vi "dfd_QMF Lattice Synthesis Bank with State (Array).vi"(6 "state in":cluster{"state":dbl[]}[](array[cluster]), 8 "error in (no error)":errorcluster, 9 "filter bank":T1 {"mBank_Type" items=["Uniform", "Non-Uniform"]; "mBank_Filters"."mMRate_SumWl" min=1 max=32 step=1; "mBank_Filters"."mMRate_InputIwl" min=1 max=32 step=1; "mBank_Filters"."mMRate_GainWl" min=1 max=32 step=1; "mBank_Filters"."mMRate_OutputWl" min=1 max=32 step=1; "mBank_Filters"."mMRate_InputWl" min=1 max=32 step=1; "mBank_Filters"."mMRate_CoefWl" min=1 max=32 step=1; "mBank_Filters"."mMRate_Mode" items=["Default"=-1, "No Rate Change"=0, "Interpolation"=1, "Decimation"=2, "Interpolated"=3, "Rational"=4]}, 10 "x 2":dbl[](array[numeric]) format="%.2f", 11 "x1":dbl[](array[numeric]) format="%.2f") -> (0 "error out":errorcluster, 3 "y1":dbl[](array[numeric]) format="%.2f", 4 "state out":cluster{dbl[]}[](array[cluster]))   [LabVIEW 2017, in "NI_DigFilter_FilterBank.lvlib"]
uses:
  <vilib>/addons/Digital Filter Design/NI_DigFilter_FilterBank.lvlib
  <vilib>/addons/Digital Filter Design/FilterBank.llb/Object/DFD Bank Obj.ctl
  <vilib>/addons/Digital Filter Design/_Objects.llb/DFD Multirate Filter Obj.ctl
  <vilib>/addons/Digital Filter Design/_Objects.llb/DFD Multirate Mode.ctl
  <vilib>/addons/Digital Filter Design/_Objects.llb/DFD Coef Norm Type.ctl
  <vilib>/addons/Digital Filter Design/_Objects.llb/DFD Round-off Mode.ctl
  <vilib>/addons/Digital Filter Design/_Objects.llb/DFD FXP MRate Multiply Mode.ctl
  <vilib>/addons/Digital Filter Design/FilterBank.llb/Object/DFD Filter Bank Processing Method.ctl
  <vilib>/addons/Digital Filter Design/FilterBank.llb/Object/DFD Filter Bank Type.ctl
  <vilib>/addons/Digital Filter Design/_Misc.llb/dfd_Error Cluster From Error Code (Scalar).vi
  <vilib>/addons/Digital Filter Design/NI_DigFilterLicensed.lvlib
  <resource>/LVDFD.dll
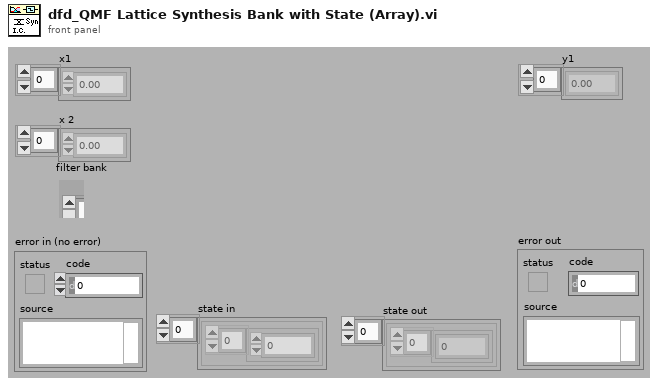
[diagram p1: front panel]
types:
  T1 = typedef "NI_DigFilter_FilterBank.lvlib/DFD Bank Obj.ctl" = cluster{"mBank_Filters":T2[], " mBank_#Bands":i32, "mBank_ProcMethod":T7, "mBank_Coeffs":dbl[], "mBank_Gain":dbl, "mBank_Type":T8}
  T2 = typedef "NI_DigFilterLicensed.lvlib/DFD Multirate Filter Obj.ctl" = cluster{"mMRate_Structure":enum16{"CIC", "FIR", "IIR", "Lattice"}, "mMRate_Mode":T3, "mMRate_Factor":i32, "mMRate_FIRParams":cluster{"mMRate_FIR_H":dbl[], "mMRate_FIR_IsNyquist?":bool, "mMRate_FIR_IsSymmetric?":bool}, "mMRate_CICParams":cluster{"mMRate_CIC_#Stage":i32, "mMRate_CIC_Lag":i32, "mMRate_CIC_Type":enum16{"Lowpass", "Highpass"}}, "mMRate_Order":i32, "mMRate_Version":string, "mMRate_Comments":string, "mMRate_RationalFactor":cluster{"mMRate_L":i32, "mMRate_M":i32}, "mMRate_Fs":dbl, "mMRate_Quantized?":bool, "mMRate_QFilterGain":dbl, "mMRate_CoefWl":i16, "mMRate_Scaling":cluster{"mMRate_ScaleByPowerOf2?":bool, "mMRate_ScaleType":T4}, "mMRate_InputWl":i16, "mMRate_OutputWl":i16, "mMRate_OutputMode":T5, "mMRate_MultMode":T6, "mMRate_BitPruning":bool, "mMRate_GainWl":i16, "mMRate_OutputFwl":i16, "mMRate_SumIwl":i16, "mMRate_InputIwl ":i16, "mMRate_SumWl":i16, "mMRate_CoefIwl":i16}
  T3 = typedef "NI_DigFilterLicensed.lvlib/DFD Multirate Mode.ctl" = i16
  T4 = typedef "NI_DigFilterLicensed.lvlib/DFD Coef Norm Type.ctl" = enum16{"No Norm", "Time Domain 1-Norm", "Time Domain 2-Norm", "Time Domain Inf-Norm"}
  T5 = typedef "NI_DigFilterLicensed.lvlib/DFD Round-off Mode.ctl" = enum16{"Nearest", "Truncation"}
  T6 = typedef "NI_DigFilterLicensed.lvlib/DFD FXP MRate Multiply Mode.ctl" = enum16{"Truncated", "Full"}
  T7 = typedef "NI_DigFilter_FilterBank.lvlib/DFD Filter Bank Processing Method.ctl" = enum16{"General", "2-Band QMF Lattice", "Cosine-Modulated"}
  T8 = typedef "NI_DigFilter_FilterBank.lvlib/DFD Filter Bank Type.ctl" = u16
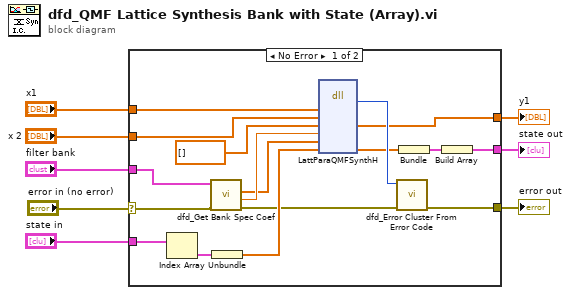
[diagram p0: block diagram]
diagram:
  n1 = case shown="No Error" "error in (no error)" {
    selector: "error in (no error)" -> [w9 w26]
    tunnel: "x1" -> [w25 _]
    tunnel: "x 2" -> [w24 _]
    tunnel: [w22 w26] -> w6
    tunnel: [w21 _] -> w5
    tunnel: "state in" -> [w18 _]
    tunnel: [w14 _] -> w3
    tunnel: "filter bank" -> [w10 _]
    frame No Error {
      n2 = Index Array(array=w18) -> (element=w19:cluster{"state":dbl[]})  [unwired: 1 in]
      n3 = call <vilib>:"dfd_Get Bank Spec Coef.vi"("error in (no error)"=w9, "bank in"=w10) -> ("error out"=w11:errorcluster, "gain"=w13:dbl, "coefficients"=w12:dbl[])  [unwired: 4 in, 3 out]
      n4 = Unbundle(w19) -> ("state"=w17:dbl[])
      n5 = dll-call lib="C:/Program Files/National Instruments/LabVIEW 2017/resource/LVDFD.*" fn="LattParaQMFSynthH"("inputDatax1H"=w25, "inputDatax2H"=w24, "outputDataH"=dbl[] [], "gainH"=w13, "coeffKH"=w12, "initialStatesH"=w17) -> ("return type"=w23:i32, "outputDataH"=w21:dbl[], "initialStatesH"=w15:dbl[])  [unwired: 7 in, 2 out]
      n6 = call-poly <vilib>:"dfd_Error Cluster From Error Code.vi"("error in (no error)"=w11, "error code (0)"=w23) -> ("error out"=w22:errorcluster)  [unwired: 9 in]
      n7 = Bundle("initialStatesH"=w15) -> (w16:cluster{"initialStatesH":dbl[]})  [unwired: 1 in]
      n8 = Build Array(w16) -> (w14:cluster{"initialStatesH":dbl[]}[])
    }
    frame Error {
    }
  }
  "error out" <- w6
  "y1" <- w5
  "state out" <- w3
